vi "S3859061_Task3.vi"() -> ()   [LabVIEW 2020]
uses:
  <vilib>/numeric/Random Number (Range) I64.vi
  <vilib>/numeric/sub_Random U32.vi
panel:
  out "y":dbl
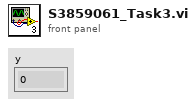
[diagram p1: front panel]
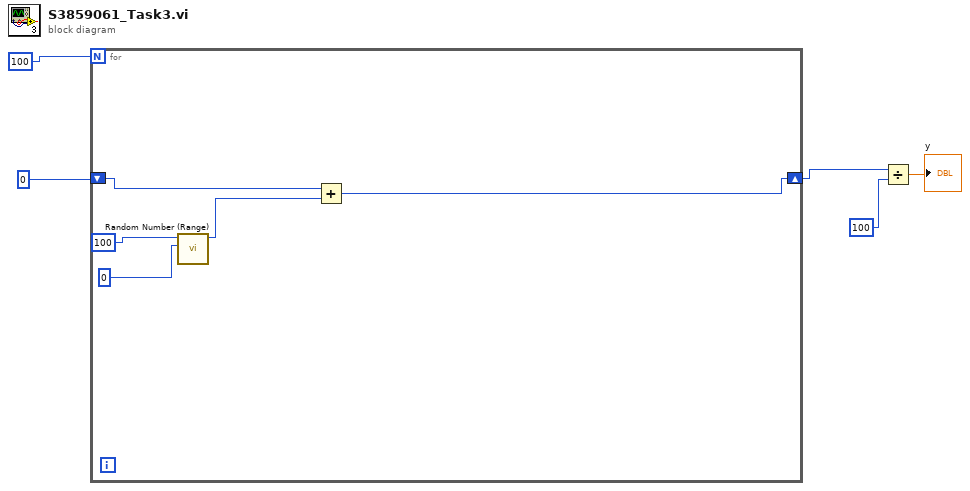
[diagram p0: block diagram]
diagram:
  n1 = for {
    N: 100 -> [_]
    shift-right: [w8] -> w3
    shift-left: 0 -> [w10]
    n2 = call-poly <vilib>:"Random Number (Range).vi"("lower bound (-100)"=0, "upper bound (100)"=100) -> ("number"=w9:i64)  [unwired: 9 in]
    n3 = Add(x=w10, y=w9) -> (x+y=w8:i64)
  }
  n4 = Divide(x=w3, y=100) -> (x/y=→"y":dbl)
